vi "connect.vi"(8 "error in (no error)":errorcluster, 11 "SerialClient in":refnum<class "SerialCommunication.lvclass">) -> (0 "error out":errorcluster, 3 "SerialClient out":refnum<class "SerialCommunication.lvclass">)   [LabVIEW 2016, in "SerialCommunication.lvclass"]
uses:
  SerialCommunication.lvclass
  SerialCommunication.lvclass/SerialCommunication.ctl
  common_serialprotocols/SerialCommunicator/SerialCommunicator.lvclass
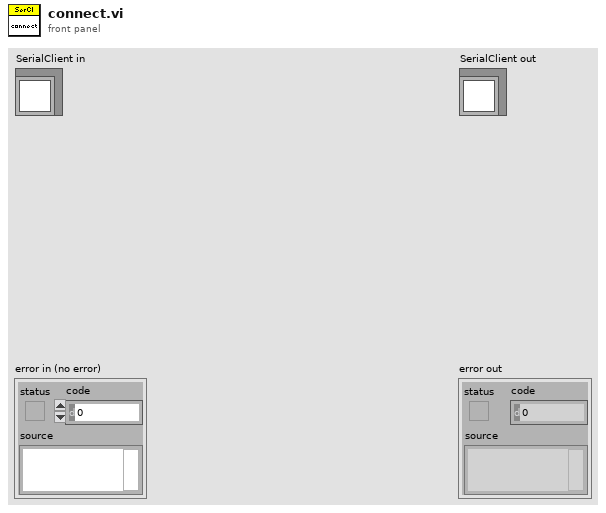
[diagram p1: front panel]
types:
  T1 = typedef "SerialProtocols.lvlib/SerialConfig.ctl" = cluster{"Serial Protocol":T2, "Protocol Parameters":T3, "Serial Message Parameters":T4}
  T2 = typedef "SerialProtocols.lvlib/SerialProtocol.ctl" = enum16{"RS232", "RS485", "SerialSimulator"}
  T3 = typedef "SerialProtocols.lvlib/ProtocolParameters.ctl" = cluster{"VISA resource name":refnum<visa-resource-name>, "Baud Rate":u32, "Data Bits":u16, "Parity":enum16{"None", "Odd", "Even", "Mark", "Space"}, "Flow Control":u16, "Stop Bits":u16, "Timeout (ms)":u32}
  T4 = typedef "SerialProtocols.lvlib/SerialMessageParameters.ctl" = cluster{"Byte Count":u32, "Enable Termination Character":bool, "Termination Char":u8}
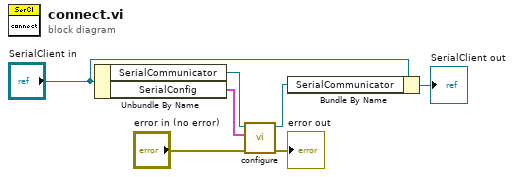
[diagram p0: block diagram]
diagram:
  n1 = Unbundle By Name("SerialClient in") -> ("SerialCommunicator"=w6:refnum<class "SerialCommunicator.lvclass">, "SerialConfig"=w7:T1)
  n2 = call-dynamic "configure.vi"("error in (no error)"="error in (no error)", "SerialConfig"=w7, "SerialCommunicator in"=w6) -> ("error out"=→"error out":errorcluster, "SerialCommunicator out"=w3:refnum<class "SerialCommunicator.lvclass">)  [unwired: 7 in]
  n3 = Bundle By Name(cluster="SerialClient in", "SerialCommunicator"=w3) -> (→"SerialClient out":refnum<class "SerialCommunication.lvclass">)
